vi "Get Result.vi"(11 "Othello":T1[][](xcontrol)) -> (3 "Resule":string)   [LabVIEW 2018]
doc: "本VI是为《我和LabVIEW》一书编写的示例。\n关于本书的介绍请参考网页：\nhttp://ruanqizhen.spaces.live.com/blog/cns!5852D4F797C53FB6!4310.entry"
uses:
  Control/Pict Ring Chess.ctl
  Othello.xctl
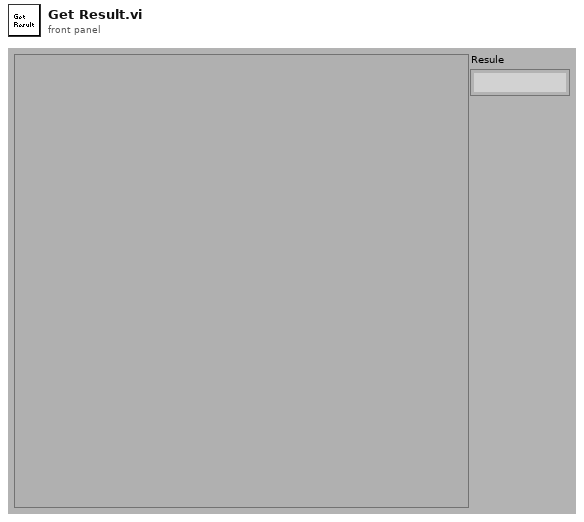
[diagram p1: front panel]
types:
  T1 = typedef "Othello.xctl/Pict Ring Chess.ctl" = u16
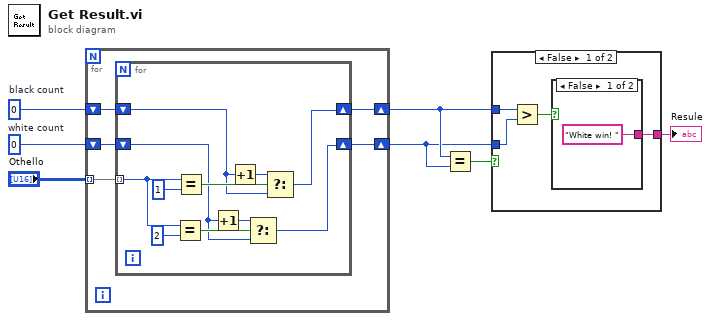
[diagram p0: block diagram]
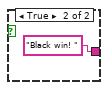
[diagram p2: hidden frame]
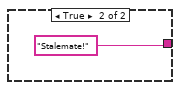
[diagram p3: hidden frame]
diagram:
  w5 = 0  # white count
  w6 = 0  # black count
  n1 = for {
    tunnel: "Othello" -> [w12] mode=indexing
    shift-right: [w9] -> w3
    shift-left: w6 -> [w11]
    shift-right: [w8] -> w2
    shift-left: w5 -> [w10]
    n2 = for {
      tunnel: w12 -> [w15] mode=indexing
      shift-right: [w19] -> w9
      shift-left: w11 -> [w20]
      shift-right: [w13] -> w8
      shift-left: w10 -> [w17]
      n3 = Equal?(x=w15, y=T1 2) -> (x = y?=w18:bool)
      n4 = Equal?(x=w15, y=T1 1) -> (x = y?=w22:bool)
      n5 = Increment(x=w17) -> (x+1=w16:i32)
      n6 = Increment(x=w20) -> (x+1=w21:i32)
      n7 = Select(t=w16, s=w18, f=w17) -> (s? t:f=w13:i32)
      n8 = Select(t=w21, s=w22, f=w20) -> (s? t:f=w19:i32)
    }
  }
  n9 = Equal?(x=w3, y=w2) -> (x = y?=w4:bool)
  n10 = case shown="False" w4 {
    tunnel: w3 -> [w27 _]
    tunnel: w2 -> [w26 _]
    tunnel: [w24 "Stalemate!"] -> w1
    frame False {
      n11 = Greater?(x=w27, y=w26) -> (0:w25:bool)
      n12 = case shown="False" w25 {
        tunnel: ["White win! " "Black win! "] -> w24
        frame False {
        }
        frame True {
        }
      }
    }
    frame True {
    }
  }
  "Resule" <- w1
